vi "PicoScope2000aClose.vi"(8 "error in (no error)":errorcluster, 11 "handle in":i16) -> (0 "error out":errorcluster, 3 "handle out":i16)   [LabVIEW 2010]
doc: "This closes the oscilloscope and should be called before exiting an application."
uses:
  ps2000a.dll
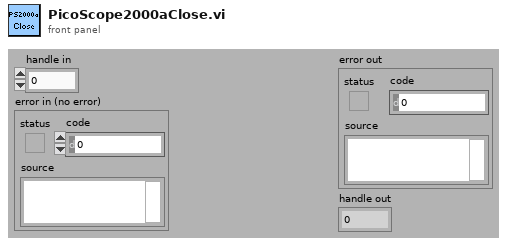
[diagram p1: front panel]
types:
  T1 = cluster{"status":bool, "code":u32, "source":string}
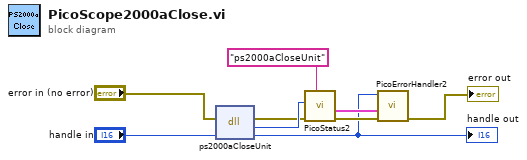
[diagram p0: block diagram]
diagram:
  n1 = dll-call lib="ps2000a.dll" fn="ps2000aCloseUnit" ("ps3000.dll:_ps3000_open_unit@0")(error in="error in (no error)", "handle"="handle in") -> (error out=w3:errorcluster, "PICO_STATUS"=w4:u32, "handle"=w5:i16)  [unwired: 2 in, 1 out]
  "handle out" <- w5
  n2 = call "PicoStatus2.vi"("PICO source"="ps2000aCloseUnit", "Error in"=w3, "PICO STATUS"=w4) -> ("error out"=w7:errorcluster, "PICO_STATUS out"=w6:T1)  [unwired: 5 in]
  n3 = call "PicoErrorHandler2.vi"("error in (no error)"=w7, "PICO_STATUS in"=w6, "handle In"=w5) -> ("error out"=→"error out":errorcluster)  [unwired: 8 in]
